vi "Multiplier 1.vi"   [LabVIEW 2010]
doc: "Little contemplated fact: This vi is actually a simple processor."
uses:
  <vilib>/rvi/DataTransferAndStorage/Container/XNode/niFpgaContainer.xnode
  <vilib>/rvi/DataTransferAndStorage/Container/Common/niFpgaContainerMetaDataKey.ctl
  <vilib>/rvi/DataTransferAndStorage/Container/Common/niFpgaContainerExecOnDevCompGetState.vi
  <vilib>/Platform/TimedLoop/XDataNode/XDataNode.xnode
  <vilib>/Platform/TimedLoop/XDataNode/nitl_modes.ctl
  <vilib>/Platform/TimedLoop/XDataNode/XDNodeRunTimeDep.lvlib
  <vilib>/Platform/TimedLoop/XDataNode/wakeup.ctl
  <vilib>/Platform/TimedLoop/XDataNode/timing_clust.ctl
  <vilib>/rvi/FXPMathLib/FxpMul/XNode/nifxpmath_Multiplier.xnode
  Motor Control Global.vi
  <vilib>/rvi/DataTransferAndStorage/Container/Common/niFpgaContainerMethod.ctl
  <vilib>/rvi/FIFO/Fifo_Types/niFpgaFifoControlLogicControl.ctl
  <vilib>/rvi/FIFO/Fifo_Resource/nirvififoEmulationSetSize.vi
  <vilib>/rvi/DataTransferAndStorage/Container/Common/niFpgaContainerGetUniqueNameForEmu.vi
  <vilib>/rvi/eio/common/nirviEmuReportErrorAndStop.vi
  <vilib>/rvi/DataTransferAndStorage/Container/Common/niFpgaTransferTypeControl.ctl
  <vilib>/rvi/interface/RandomDataEmulation/nirviRandomDataFPGAFIFO.vi
  <vilib>/rvi/interface/RandomDataEmulation/niFpgaRandomDataHandleErrors.vi
  <vilib>/rvi/DataTransferAndStorage/FIFO/niFpgaPeerToPeerStreamState.ctl
  <vilib>/rvi/FXPMathLib/FxpMul/simVIs/DllFxpMulTemp_sub.vi
  <vilib>/fxp/LVFixedPointOverflowPolicyTypeDef.ctl
  <vilib>/fxp/LVFixedPointQuantizationPolicyTypeDef.ctl
  <vilib>/rvi/FXPMathLib/FxpMul/subVIs/nifxpmath_Mul_SimConfig.ctl
  <vilib>/rvi/Memory/Memory_Emulation/nirvimemoryEmulationManagerCache_GetValue.vi
  <vilib>/rvi/Memory/Memory_Emulation/nirvimemoryEmulationManagerCache_InsertValue.vi
  <vilib>/Utility/error.llb/Clear Errors.vi
  <vilib>/rvi/Memory/Memory_Emulation/nirvimemoryEmulationManagerCache_SetValue.vi
types:
  T1 = typedef "niFpgaContainerMetaDataKey.ctl" = enum16{"FPGA FIFO", "FPGA Memory", "FPGA Register"}
  T2 = typedef "niFpgaFifoControlLogicControl.ctl" = enum16{"Slice Fabric", "Target Optimal", "Built-in"}
  T3 = typedef "niFpgaContainerMethod.ctl" = enum16{"<none>", "write", "read", "clear", "getNumberOfElementsToWrite", "getNumberOfElementsToRead", "enable", "disable", "flushAndDisable", "getStreamState", "readA", "readB", "dramWrite", "dramWriteWithByteEnables", "dramRequestData", "dramRetrieveData"}
  T4 = typedef "niFpgaTransferTypeControl.ctl" = enum16{"Target-Scoped", "Host to Target - DMA", "Target to Host - DMA", "Peer to Peer Reader", "Peer to Peer Writer", "Bidirectional"}
  T5 = typedef "niFpgaPeerToPeerStreamState.ctl" = enum16{"Unlinked", "Disabled", "Enabled", "Flushing"}
  T6 = typedef "XDNodeRunTimeDep.lvlib/timing_clust.ctl" = cluster{"Expected End [f-1]":u64, "Actual End [f-1]":u64, "Finished Late? [f-1]":bool, "Expected End [i-1]":u64, "Actual End [i-1]":u64, "Finished Late? [i-1]":bool, "Expected Start [i]":u64, "Actual Start [i]":u64, "Expected Start [f]":u64, "Actual Start [f]":u64, "Source Name":string, "Structure Name":string, "Period":i64, "Deadline":i64, "Offset":i64, "Start":i64, "Priority":i32, "Timeout":i32, "Mode":T7, "Wakeup Reason":T8, "Error":errorcluster, "Source Type":string, "Secondary Source Type":string, "Global End Time":u64, "Global Start Time":u64, "Frame Duration":u64, "Iteration Duration":u64, "Assigned CPU":i32, "I/O Scan Engine Mode":u32}
  T7 = typedef "XDNodeRunTimeDep.lvlib/nitl_modes.ctl" = enum32{"No Change", "Process missed periods, maintain original phase", "Discard missed periods, maintain original phase", "Process missed periods, ignore original phase", "Discard missed periods, ignore original phase"}
  T8 = typedef "XDNodeRunTimeDep.lvlib/wakeup.ctl" = enum32{"Normal", "Aborted", "Asynchronous wakeup", "Timing source error", "Timed loop error", "Timeout"}
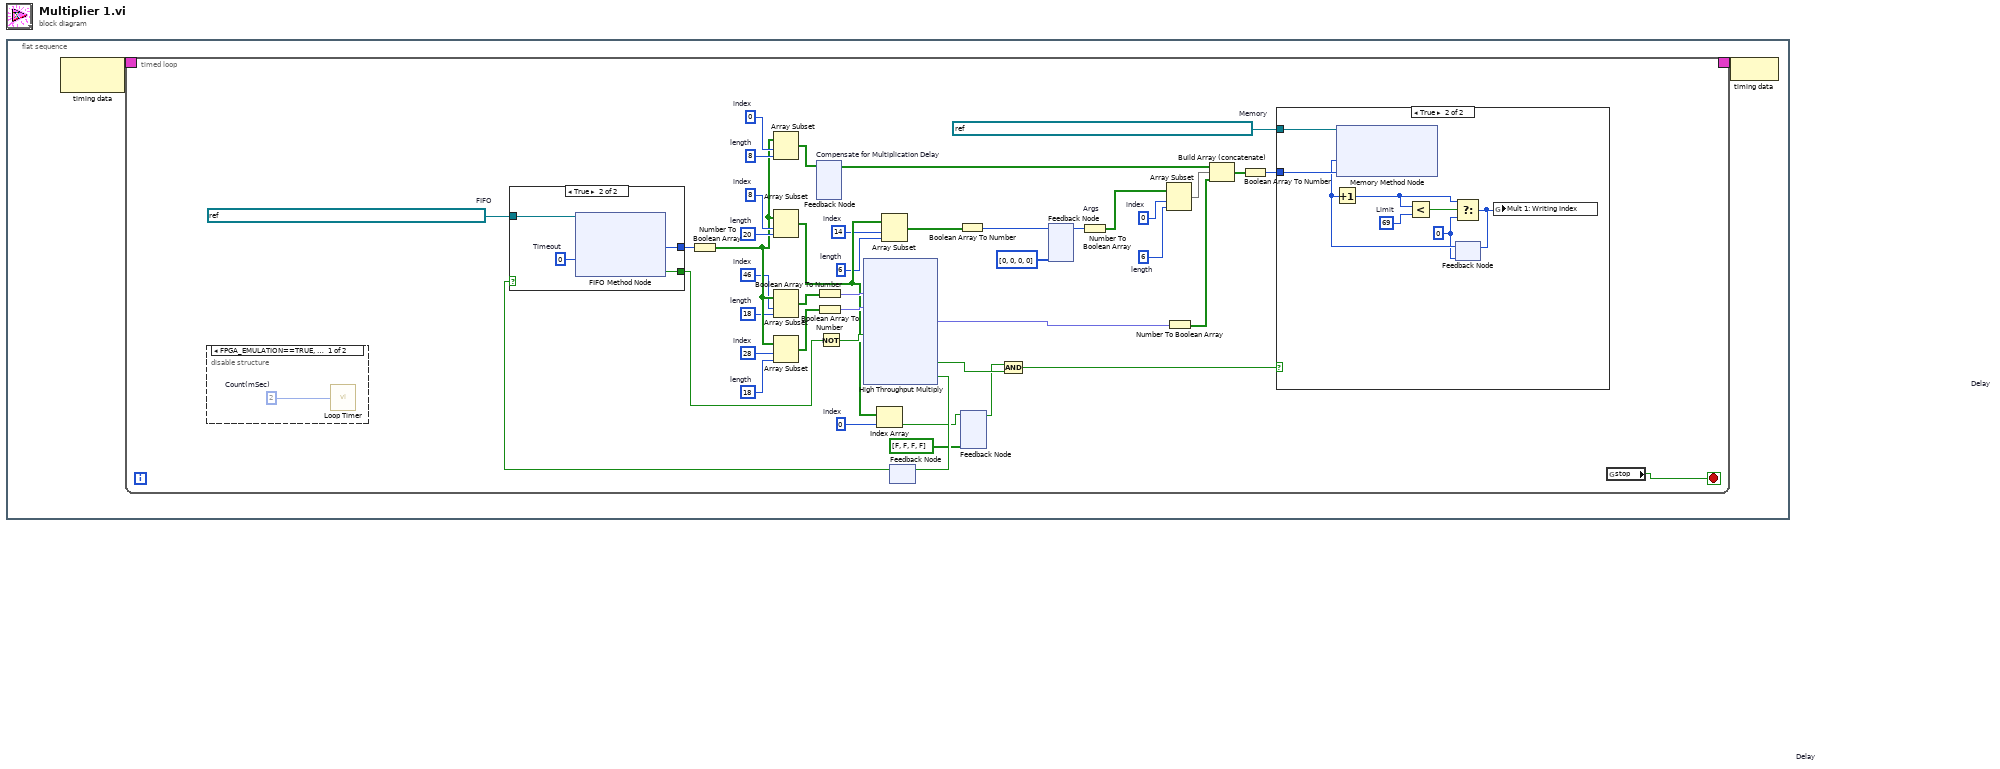
[diagram p0: block diagram]
diagram:
  n1 = flat-sequence {
    frame #0 {
      n2 = node-c288() -> (w2:T6)  [unwired: 1 in]
      n3 = timed-loop {
        timing: w2 -> [_]
        timing-out: [_] -> w1
        stop <- w19 stop-if-true
        w4 = refnum<k21> "Multiplier 1 FIFO In :  [8b Idendifier; 20b args; 18b fxp ; 18b fxp]"  # FIFO
        w3 = refnum<k21> "Multiplier 1 Block Memory Out : [8b Identifier; 6b args; 18b fxp output]"  # Memory
        w5 = 6  # length
        w6 = 0  # index
        w13 = 6  # length
        w14 = 14  # index
        w21 = 0  # index
        w35 = 18  # length
        w36 = 46  # index
        w38 = 18  # length
        w39 = 28  # index
        w40 = 20  # length
        w41 = 8  # index
        w42 = 8  # length
        w43 = 0  # index
        n4 = disable-structure shown="FPGA_EMULATION==TRUE, default" {
          frame condition #0 {
            w47 = u32 2  # Count(mSec)
            n5 = call "Loop Timer"("Count(mSec)"=w47) -> ()  [unwired: 1 out]
          }
          frame condition #1 (active) {
          }
        }
        n6 = feedback #1 "Compensate for Multiplication Delay"() -> (w22:bool[])  [unwired: 1 in]
        n7 = feedback #2() -> (w26:bool)  [unwired: 1 in]
        n8 = case shown="True" w26 {
          tunnel: w4 -> [_ w255]
          tunnel: [_ w254] -> w46
          tunnel: [_ w253] -> w44
          frame False {
          }
          frame True {
            w252 = 0  # Timeout
            n9 = xnode ("FIFO Method Node")("Timeout"=w252, "FIFO In"=w255) -> ("Element"=w253:u64, "Timed Out?"=w254:bool)  [unwired: 1 out]
          }
        }
        n10 = Number To Boolean Array(number=w44) -> (Boolean array=w37:bool[])
        n11 = Array Subset(array=w37, index=w43, length=w42) -> (w30:bool[])
        n12 = Array Subset(array=w37, index=w41, length=w40) -> (w15:bool[])
        n13 = Array Subset(array=w37, index=w36, length=w35) -> (w34:bool[])
        n14 = Array Subset(array=w37, index=w39, length=w38) -> (w33:bool[])
        n15 = feedback-in #1(w30) -> ()
        n16 = Boolean Array To Number(Boolean array=w34) -> (number=w24:fxp<+/-,18,1>)
        n17 = Boolean Array To Number(Boolean array=w33) -> (number=w23:fxp<+/-,18,1>)
        n18 = Not(x=w46) -> (.not. x?=w45:bool)
        n19 = xnode "High Throughput Multiply"("x"=w24, "y"=w23, "input valid"=w45) -> ("x*y"=w32:fxp<+/-,18,1>, "output valid"=w25:bool, "ready for input"=w27:bool)  [unwired: 1 in]
        n20 = Index Array(array=w15, index=w21) -> (element=w18:bool)
        n21 = Array Subset(array=w15, index=w14, length=w13) -> (w12:bool[])
        n22 = feedback-in #2(w27) -> ()
        n23 = Boolean Array To Number(Boolean array=w12) -> (number=w11:u8)
        n24 = feedback-in #3(w18) -> ()
        n25 = feedback #3 "Delay"(bool[] [FALSE, FALSE, FALSE, FALSE]) -> (w17:bool)
        n26 = And(x=w17, y=w25) -> (x .and. y?=w20:bool)
        n27 = feedback-in #4(w11) -> ()
        n28 = feedback #4 "Delay"(u8[] [0, 0, 0, 0]) -> (w9:u8)
        n29 = Number To Boolean Array "Args"(number=w9) -> (Boolean array=w8:bool[])
        n30 = Array Subset(array=w8, index=w6, length=w5) -> (w7:bool[])
        n31 = Number To Boolean Array(number=w32) -> (Boolean array=w29:bool[])
        n32 = Build Array (concatenate)(w22, w7, w29) -> (w31:bool[])
        n33 = Boolean Array To Number(Boolean array=w31) -> (number=w28:u32)
        n34 = case shown="True" w20 {
          tunnel: w3 -> [_ w55]
          tunnel: w28 -> [_ w51]
          frame False {
          }
          frame True {
            w53 = u32 69  # Limit
            w48 = u32 0
            n35 = feedback #5(w48) -> (w50:u32)
            n36 = Increment(x=w50) -> (x+1=w54:u32)
            n37 = xnode ("Memory Method Node")("Address"=w50, "Data"=w51, "Memory In"=w55) -> ()  [unwired: 1 out]
            n38 = Less?(x=w54, y=w53) -> (x < y?=w52:bool)
            n39 = Select(t=w54, s=w52, f=w48) -> (s? t:f=w49:u32)
            n40 = feedback-in #5(w49) -> ()
            n41 = global write "Motor Control Global.vi" "Mult 1: Writing Index"(w49) -> ()
          }
        }
        n42 = global read "Motor Control Global.vi" "stop"() -> (w19:bool)
      }
      n43 = node-c288(w1) -> ()
    }
  }
